vi "Data.vi"(10 "Channel select":tag, 11 "Acceleration in\nm/s^2    or    g":bool) -> (3 "Data":dbl)   [LabVIEW 2019]
uses:
  <vilib>/DAQmx/read.llb/DAQmx Read (Analog DBL 1Chan 1Samp).vi
  <vilib>/DAQmx/create/channels.llb/DAQmx Create Channel (AI-Voltage-Basic).vi
  <vilib>/DAQmx/miscellaneous.llb/DAQmx Fill In Error Info.vi
panel:
  out "Numeric 2":dbl
  out "Numeric":dbl
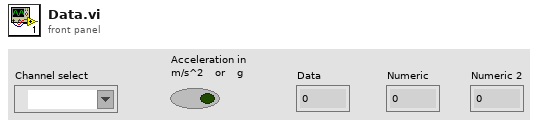
[diagram p1: front panel]
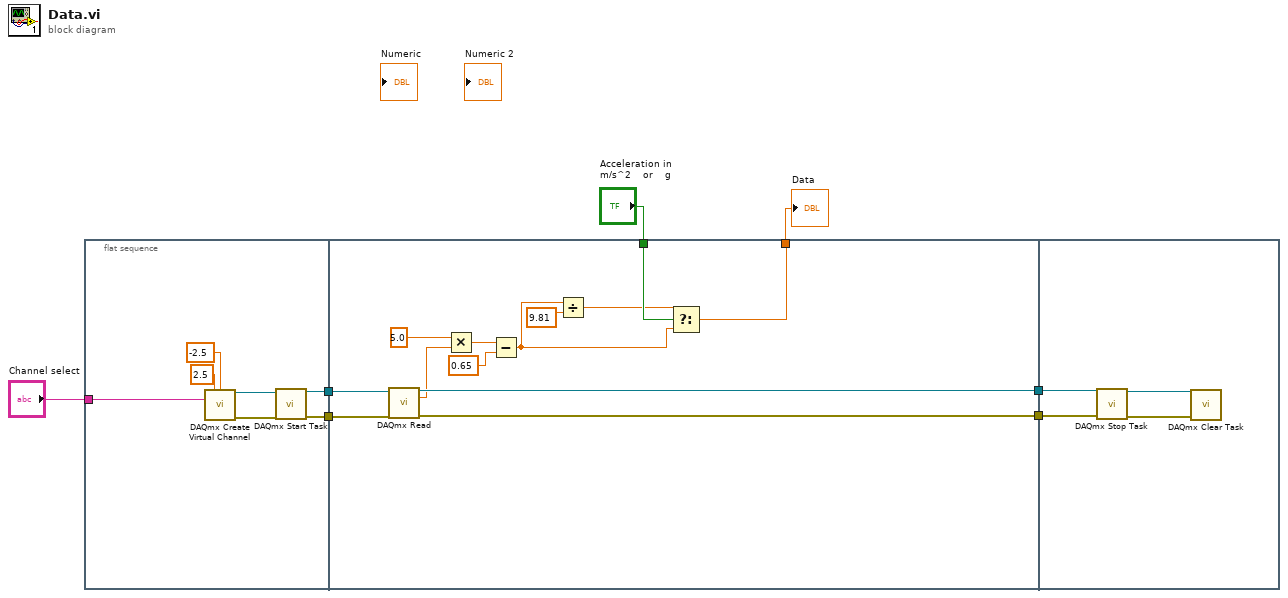
[diagram p0: block diagram]
diagram:
  n1 = flat-sequence {
    tunnel: [w11] -> w7
    tunnel: [w9] -> w6
    tunnel: "Channel select" -> [w8]
    tunnel: w7 -> [w27]
    tunnel: w6 -> [w26]
    tunnel: [w25] -> w5
    tunnel: [w24] -> w4
    tunnel: [w23] -> w3
    tunnel: "Acceleration in\nm/s^2    or    g" -> [w22]
    tunnel: w5 -> [w28]
    tunnel: w4 -> [w31]
    frame #0 {
      n2 = call-poly <vilib>:"DAQmx Create Virtual Channel.vi"("maximum value"=2.5, "minimum value"=-2.5, "physical channels"=w8) -> ("task out"=w12:refnum<k21>, "error out"=w10:errorcluster)  [unwired: 11 in]
      n3 = call <vilib>:"DAQmx Start Task.vi"("task/channels in"=w12, "error in"=w10) -> ("task out"=w11:refnum<k21>, "error out"=w9:errorcluster)  [unwired: 12 in]
    }
    frame #1 {
      n4 = call-poly <vilib>:"DAQmx Read.vi"("task/channels in"=w27, "error in"=w26) -> ("task out"=w24:refnum<k21>, "data"=w17:dbl, "error out"=w25:errorcluster)  [unwired: 11 in]
      n5 = Multiply(x=5.0, y=w17) -> (x*y=w18:dbl)
      n6 = Subtract(x=w18, y=0.65) -> (x-y=w20:dbl)
      n7 = Divide(x=w20, y=9.81) -> (x/y=w21:dbl)
      n8 = Select(t=w21, s=w22, f=w20) -> (s? t:f=w23:dbl)
    }
    frame #2 {
      n9 = call <vilib>:"DAQmx Stop Task.vi"("task/channels in"=w31, "error in"=w28) -> ("task out"=w30:refnum<k21>, "error out"=w29:errorcluster)  [unwired: 12 in]
      n10 = call <vilib>:"DAQmx Clear Task.vi"("task in"=w30, "error in"=w29) -> ()  [unwired: 13 in, 1 out]
    }
  }
  "Data" <- w3
